vi "OFDM-SIM信号生成.vi"(0 "总比特数":i32=2500, 1 "载波数":i32=125, 2 "M-QAM":i32=4 caption="M-QAM (16)", 3 "error in (no error)":errorcluster) -> (4 "输入比特流":i8[](array[numeric]) caption="output bit stream", 5 "并行信号":cdb[][](array[numeric]), 6 "理论4QAM星座图":cdb[](graph), 7 "比特/符号":i32 caption="bits per symbol", 8 "error out":errorcluster)   [LabVIEW 2018]
uses:
  <vilib>/addons/Modulation/Digital/General/MT Generate Bits (Galois, PN Order).vi
  <vilib>/addons/Modulation/Digital/Support/Common/Validators/mod_Generate Bits Validate.vi
  <vilib>/addons/Modulation/Analog/support/mod_Set Error Source.vi
  <vilib>/addons/Modulation/Digital/General/MT Generate QAM System Parameters(M).vi
  <vilib>/addons/Modulation/Digital/General/subVIs/mod_Generate Bits PN Sequence.vi
  <vilib>/addons/Modulation/Digital/General/MT Map Bits to QAM Symbols.vi
  <vilib>/addons/Modulation/niDMT.lvlib
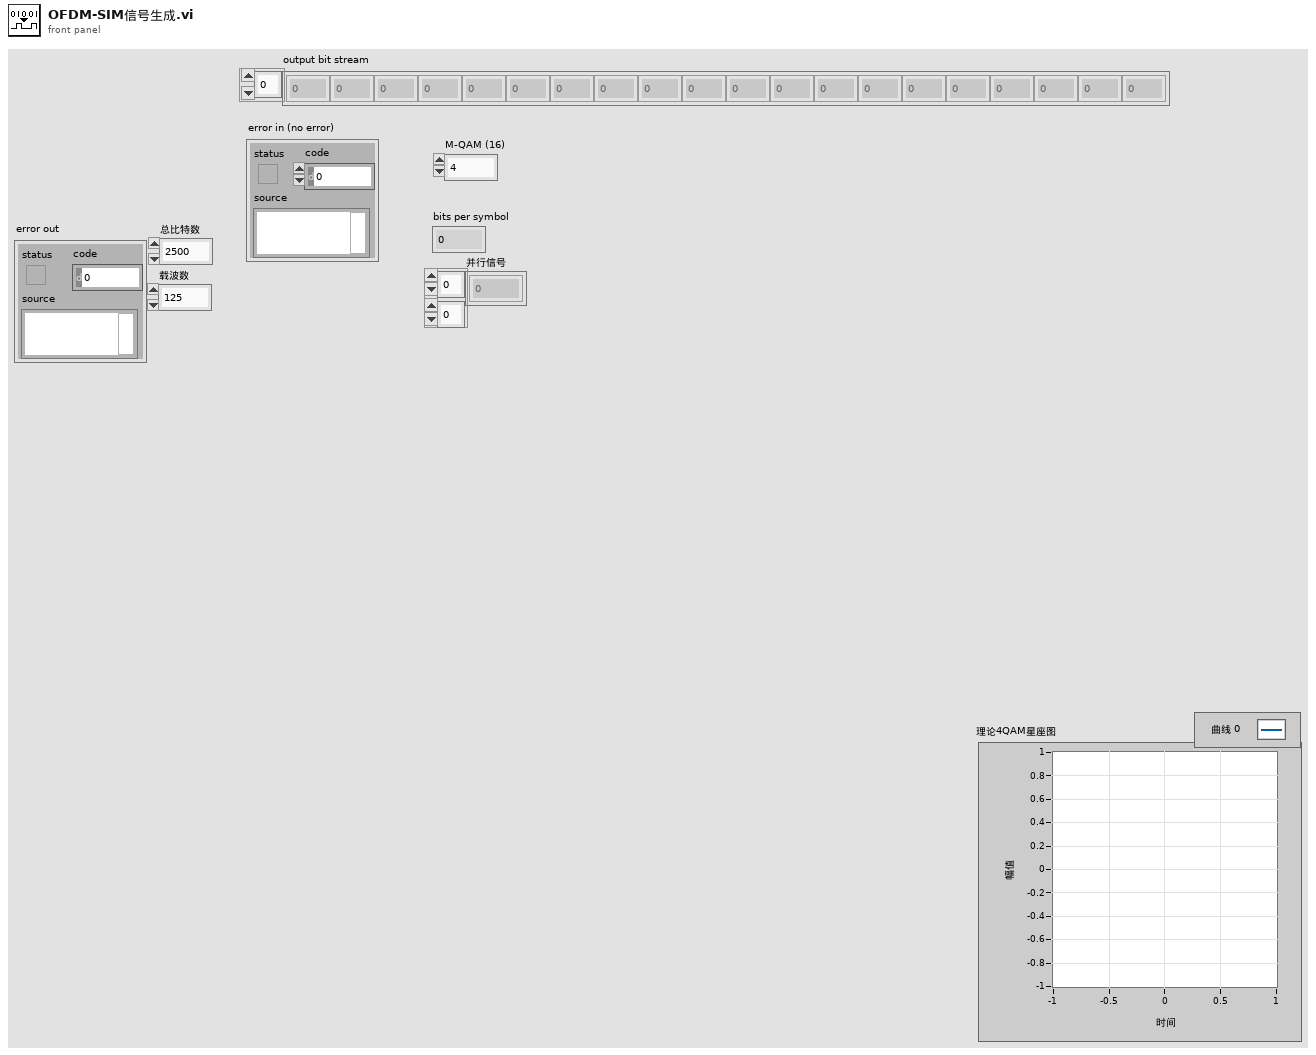
[diagram p1: front panel]
types:
  T1 = cluster{"samples per symbol (16)":i32, "symbol map":cdb[]}
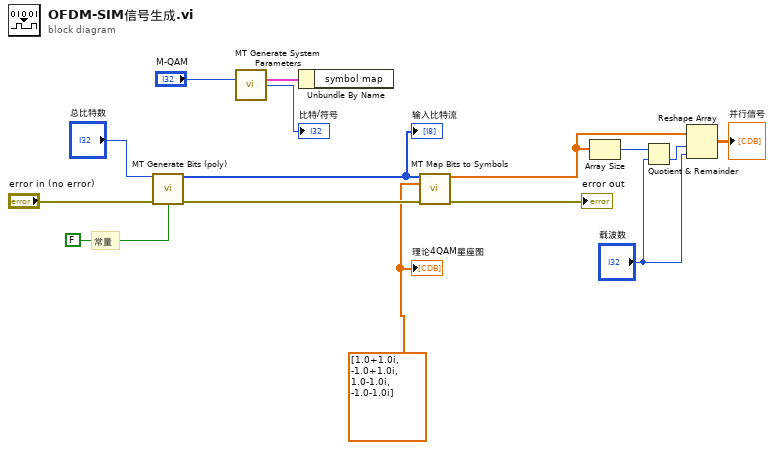
[diagram p0: block diagram]
diagram:
  w1 = cdb[] [1.0+1.0i, -1.0+1.0i, 1.0-1.0i, -1.0-1.0i]
  # "常量"
  n1 = call-poly <vilib>:"MT Generate Bits (poly).vi"("total bits (128)"="总比特数", "error in (no error)"="error in (no error)", "reset? (T)"=FALSE) -> ("output bit stream"=w4:i8[], "error out"=w13:errorcluster)  [unwired: 10 in, 1 out]
  "输入比特流" <- w4
  n2 = call-poly <vilib>:"MT Generate System Parameters.vi"("M-QAM (16)"="M-QAM") -> ("QAM system parameters"=w6:T1, "bits per symbol"=→"比特/符号":i32)  [unwired: 12 in, 1 out]
  n3 = Unbundle By Name(w6) -> ()  [unwired: 1 out]
  n4 = call-poly <vilib>:"MT Map Bits to Symbols.vi"("input bit stream"=w4, "symbol map"=w1, "error in (no error)"=w13) -> ("symbols"=w5:cdb[], "error out"=→"error out":errorcluster)  [unwired: 11 in]
  n5 = Array Size(array=w5) -> (size(s)=w11:i32)
  n6 = Quotient & Remainder(x=w11, y="载波数") -> (floor(x/y)=w10:i32)  [unwired: 1 out]
  n7 = Reshape Array ("重排数组维数")(w5, w10, "载波数") -> (→"并行信号":cdb[][])
  "理论4QAM星座图" <- w1
